vi "ClassAttributes_ReadClassAttributes_4x4x4_Singleton.vi"(8 "error in (no error)":errorcluster) -> (0 "error out":errorcluster)   [LabVIEW 2010]
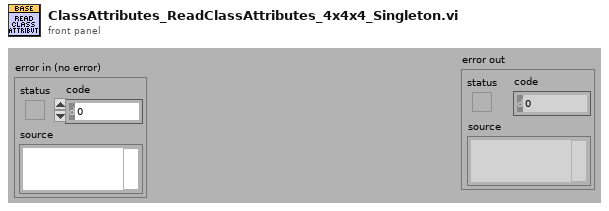
[diagram p1: front panel]
types:
  T1 = typedef "ClassAttributes_ClassAttributes.ctl" = cluster{"classAttribute1":bool}
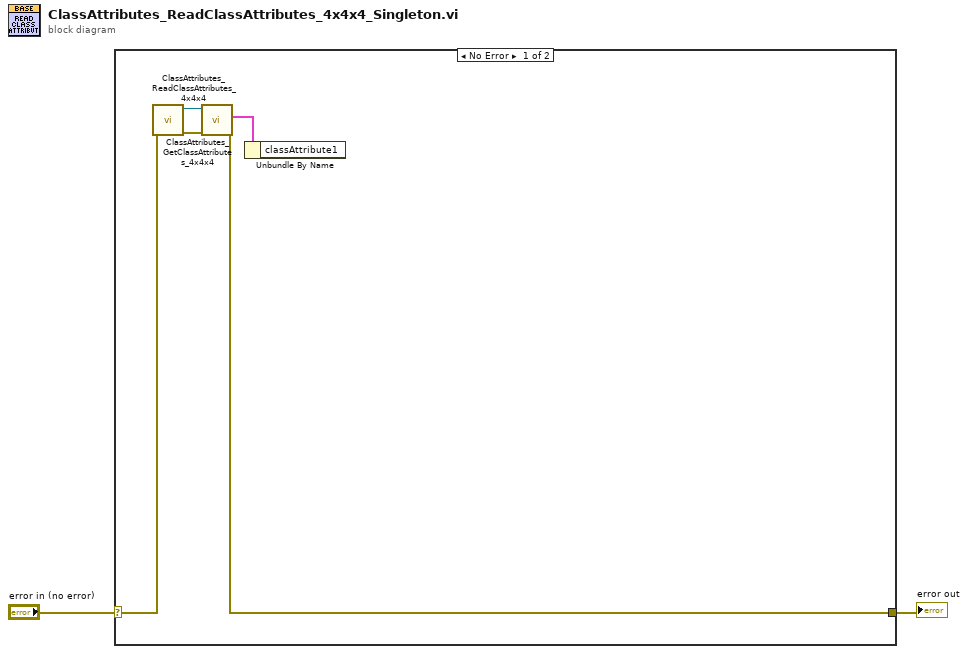
[diagram p0: block diagram]
diagram:
  n1 = case shown="No Error" "error in (no error)" {
    selector: "error in (no error)" -> [w4 w8]
    tunnel: [w6 w8] -> w1
    frame No Error {
      n2 = call "ClassAttributes_ReadClassAttributes_4x4x4.vi"("error in (no error)"=w4) -> ("error out"=w3:errorcluster, "reference out"=w5:refnum<class>)  [unwired: 9 in]
      n3 = call "ClassAttributes_GetClassAttributes_4x4x4.vi"("error in (no error)"=w3, "reference in"=w5) -> ("error out"=w6:errorcluster, "Class attribute"=w7:T1)  [unwired: 6 in, 2 out]
      n4 = Unbundle By Name(w7) -> ()  [unwired: 1 out]
    }
    frame Error {
    }
  }
  "error out" <- w1
